vi "Main.vi"(11 "Module Admin":refnum<class "Delacor_lib_QMH_Module Admin.lvclass">) -> ()   [LabVIEW 2024, in "UI.lvlib"]
doc: "This template is based off of the Queued Message Handler design pattern and the Queued Message Handler project template that ships with LabVIEW.\n\nThe main difference is that the queue is private to this module and communication between modules is performed via Broadcast and Request events.\n\nRequest events are wrapped in public API methods and are handled in the Event Handling Loop (EHL) of this VI. Any module can register for Broadcast events sent by this module. The EHL generates messages based on user interface actions.\n\nThe Message Handling Loop (MHL) processes messages generated by the EHL, or by other messages. The messages are string values, so new messages can be added easily to the Message Cases case structure in the MHL. Each message cluster can also provide an optional value for Message Data, which is a variant that can be converted to whatever message-specific data is required.\n_____\nBased on DQMH Project Template 7.0.0.1280."
uses:
  UI.lvlib
  <vilib>/Delacor/Delacor QMH/Libraries/Module Admin_class/Delacor_lib_QMH_Module Admin.lvclass
  Module Data--cluster.ctl
  Ready Drive State Machine.ctl
  Start Ready Drive State Machine (Reply Payload)--cluster.ctl
  <vilib>/Delacor/Delacor QMH/Libraries/Message Queue_class/Delacor_lib_QMH_Message Queue.lvclass/Delacor_lib_QMH_Message Queue.ctl
  Stop Argument--cluster.ctl
  <vilib>/Delacor/Delacor QMH/Libraries/Module Admin_class/Delacor_lib_QMH_Module Admin.lvclass/Delacor_lib_QMH_Module Admin.ctl
  <vilib>/Utility/miscctls.llb/LVPointTypeDef.ctl
  <vilib>/Delacor/Delacor QMH/Libraries/Message Queue_class/Delacor_lib_QMH_Enqueue Message (Single).vi
  <vilib>/Delacor/Delacor QMH/Libraries/Module Admin_class/Delacor_lib_QMH_Get External Launch.vi
  <vilib>/Delacor/Delacor QMH/Libraries/Message Queue_class/Delacor_lib_QMH_Message Queue.lvclass
  Hardware Controller/Hardware Controller.lvlib
  Logger/Logger.lvlib
  Auto Mode/Auto Modo.lvlib
panel:
  in  "Fault Tab Control":enum32{"System Fault"}(tab)
  out "System Fault":bool
  in  "Clear Fault":bool
  in  "Data Tab Control":enum32{"XFL Data"}(tab)
  out "Pump Current RPM":dbl(knob) scale=0.0..1600.0
  out "Turbine Current RPM":dbl(knob) scale=0.0..1600.0 scale format="%#.3g"
  out "Turbine Shaft Torque (Nm)":dbl(knob) scale=0.0..25.0 scale format="%#.3g"
  out "Flow Velocity (m/s)":dbl(knob) scale=0.0..3.0
  out "Temperature (°C)":dbl(knob) scale=10.0..40.0
  out "Pressure Turbine Outlet":dbl(knob) scale=0.0..10.0
  out "Pressure Turbine Inlet":dbl(knob) scale=0.0..10.0
  out "Pressure Pump Outlet":dbl(knob) scale=0.0..10.0
  out "Pressure Pump Inlet":dbl(knob) scale=0.0..10.0
  in  "Logger Tab Control":enum32{"Logger"}(tab)
  in  "Start Logging":bool
  in  "Stop Logging":bool
  in  "Folder Path":path
  out "Logging":bool
  in  "Auto Mode Tab Control":enum32{"Auto Mode"}(tab)
  out "Total Steps":i32
  in  "Start Sequence":bool
  in  "Auto Configuration File":path
  in  "Load Configuration":bool
  out "Pump RPMs":i64[](array[numeric])
  out "Turbine RPMs":i64[](array[numeric])
  out "Duration":i64[](array[numeric])
  out "Current Step":i32
  out "Auto Mode Status":bool
  out "Steps Slide":dbl(slide) scale=0.0..10.0
  out "IOLink System State Out":map{string, dbl}(c390)
  in  "IOLink Connections Tab":enum32{"IOLink Connection"}(tab)
  in  "Close IOLink Connection":bool
  in  "Start IOLink Connection":bool
  out "IOLink Connection Status":bool
  out "error out":errorcluster
  in  "Drive Manual Control":enum32{"Drive Manual Control"}(tab)
  in  "Set Turbine RPM":bool
  out "Pump Ready":bool
  out "Turbine Ready":bool
  out "Pump Actual RPM":dbl
  out "Turbine Actual RPM":dbl
  in  "Pump Target RPM":i16
  in  "Turbine Target RPM":i16
  in  "Set Pump RPM":bool
  in  "Set Both RPM":bool
  in  "Set Ready":bool
  in  "EtherCAT Connections":enum32{"EtherCAT Connections"}(tab)
  out "Attempt EtherCAT Connection":bool
  out "EtherCAT Connection Status":bool
  in  "Start EtherCAT Connection":bool
  in  "Close EtherCAT Connection":bool
  in  "Abort":bool
  out "EtherCAT System State Out":map{string, dbl}(c390)
  out "Status":string
  in  "Simulate MHL Error":bool
  in  "Simulate EHL Error":bool
  # "This template is for the DQMH framework. See the block diagram for more information on how to use this template."
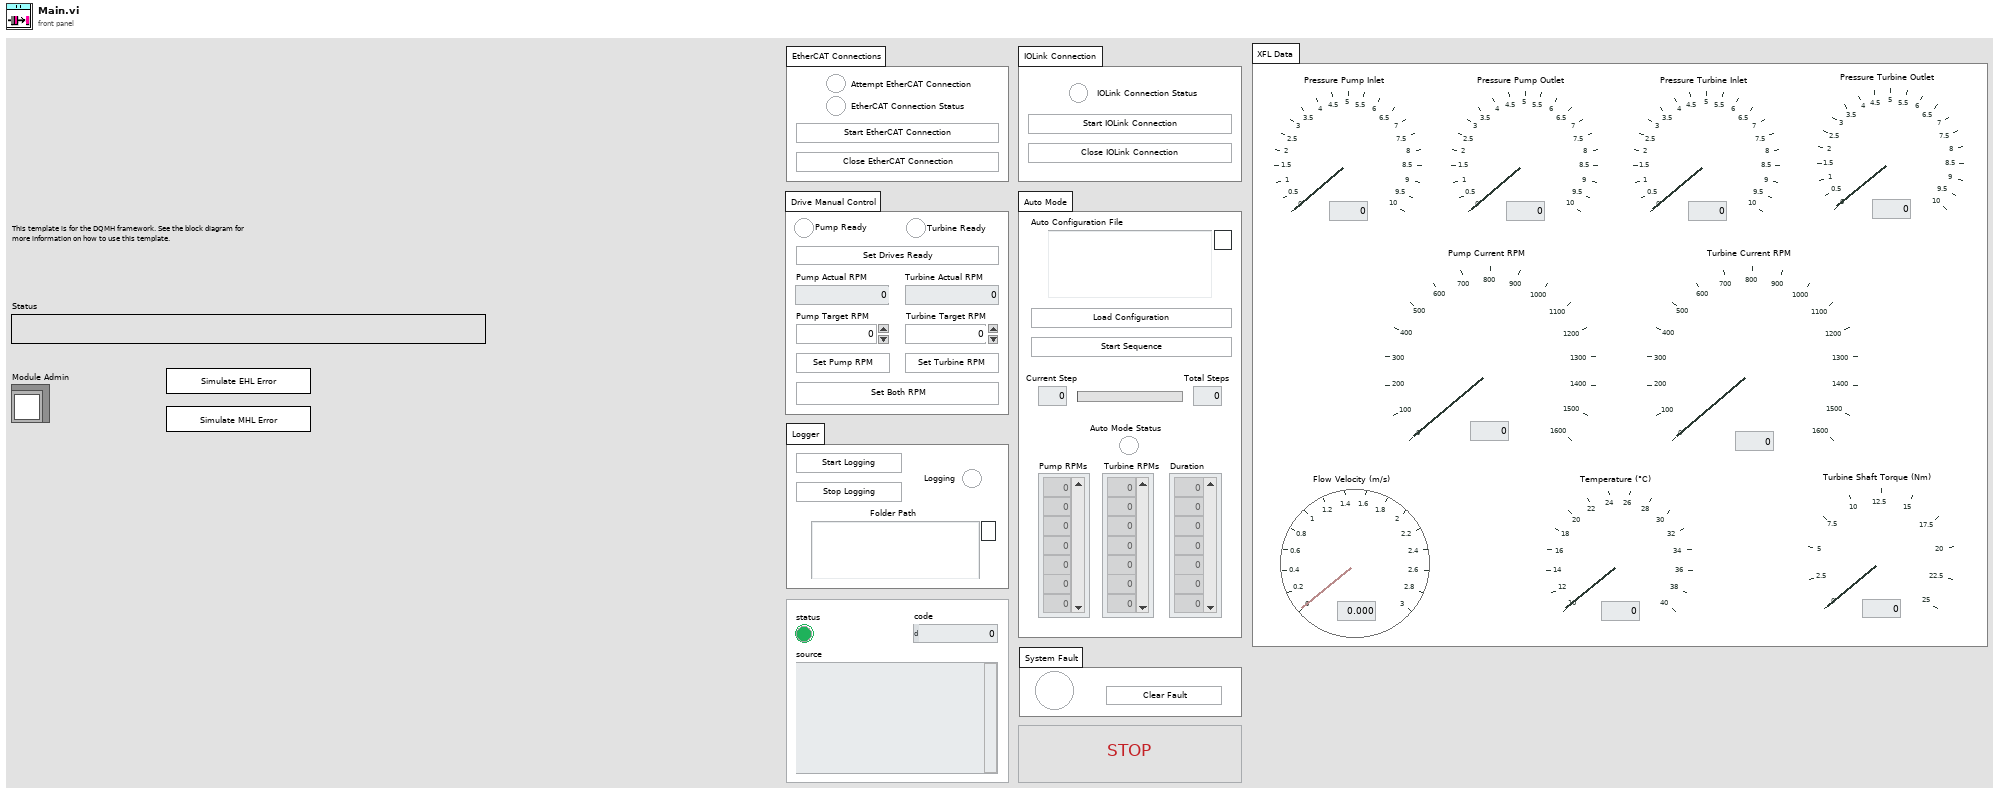
[diagram p1: front panel]
types:
  T1 = typedef "UI.lvlib/Request Events--cluster.ctl" = cluster{"Stop Module":refnum<user-event>, "Show Panel":refnum<user-event>, "Hide Panel":refnum<user-event>, "Get Module Execution Status":refnum<user-event>, "Show Diagram":refnum<user-event>, "Private":cluster{"Launch Hardware Controller":refnum<user-event>, "Register Helper Loop for Hardware Contrller Broadcast":refnum<user-event>, "Start Logger Module":refnum<user-event>, "Start Auto Mode Module":refnum<user-event>}, "Start Ready Drive State Machine":refnum<user-event>}
  T2 = typedef "Logger.lvlib/Broadcast Events--cluster.ctl" = cluster{"Module Did Init":refnum<user-event>, "Status Updated":refnum<user-event>, "Error Reported":refnum<user-event>, "Module Did Stop":refnum<user-event>, "Update Module Execution Status":refnum<user-event>, "Logger Status Updated":refnum<user-event>}
  T3 = typedef "Auto Modo.lvlib/Broadcast Events--cluster.ctl" = cluster{"Module Did Init":refnum<user-event>, "Status Updated":refnum<user-event>, "Error Reported":refnum<user-event>, "Module Did Stop":refnum<user-event>, "Update Module Execution Status":refnum<user-event>, "Current RPM Index":refnum<user-event>, "Auto Mode Status Updated":refnum<user-event>}
  T4 = typedef "Hardware Controller.lvlib/Broadcast Events--cluster.ctl" = cluster{"Module Did Init":refnum<user-event>, "Status Updated":refnum<user-event>, "Error Reported":refnum<user-event>, "Module Did Stop":refnum<user-event>, "Update Module Execution Status":refnum<user-event>, "System State Updated":refnum<user-event>, "EtherCAT Data Updated":refnum<user-event>, "System Fault Updated":refnum<user-event>, "EtherCAT Connection Status Updated":refnum<user-event>, "HardwareController IOLink Data Updated":refnum<user-event>, "IOLink Connection Updated":refnum<user-event>, "HardwareController EtherCAT Data Updated":refnum<user-event>}
  T5 = typedef "UI.lvlib/Ready Drive State Machine.ctl" = cluster{"Wait Notifier":refnum<notifier>, "wait for reply":bool, "Timeout":i32, "State":enum16{"Clear Fault", "Check Fault", "Set Ready to Switch ON", "Check Ready to Switch ON", "Set Switch ON", "Check Switch ON", "Ready Drive Completed"}, "Error":errorcluster}
  T6 = typedef "UI.lvlib/Module Data--cluster.ctl" = cluster{"Status":string, "Pump RPMs":i64[], "Duration":i64[], "Turbine RPMs":i64[]}
  T7 = enum16{"Clear Fault", "Check Fault", "Set Ready to Switch ON", "Check Ready to Switch ON", "Set Switch ON", "Check Switch ON", "Ready Drive Completed"}
  T8 = typedef "UI.lvlib/Start Ready Drive State Machine (Reply Payload)--cluster.ctl" = cluster{"error":errorcluster}
  T9 = enum32{"invalid lock state", "Not Locked", "Locked (No Password)", "Password-protected"}
  T10 = typedef "UI.lvlib/Stop Argument--cluster.ctl" = cluster{"Origin":string, "Exit via Stop Module Req?":bool, "Wait for Module to stop?":bool}
  T11 = typedef "LVPointTypeDef.ctl" = cluster{"Horizontal":i16, "Vertical":i16}
  T12 = enum32{"Invalid", "Standard", "Closed", "Hidden", "Minimized", "Maximized"}
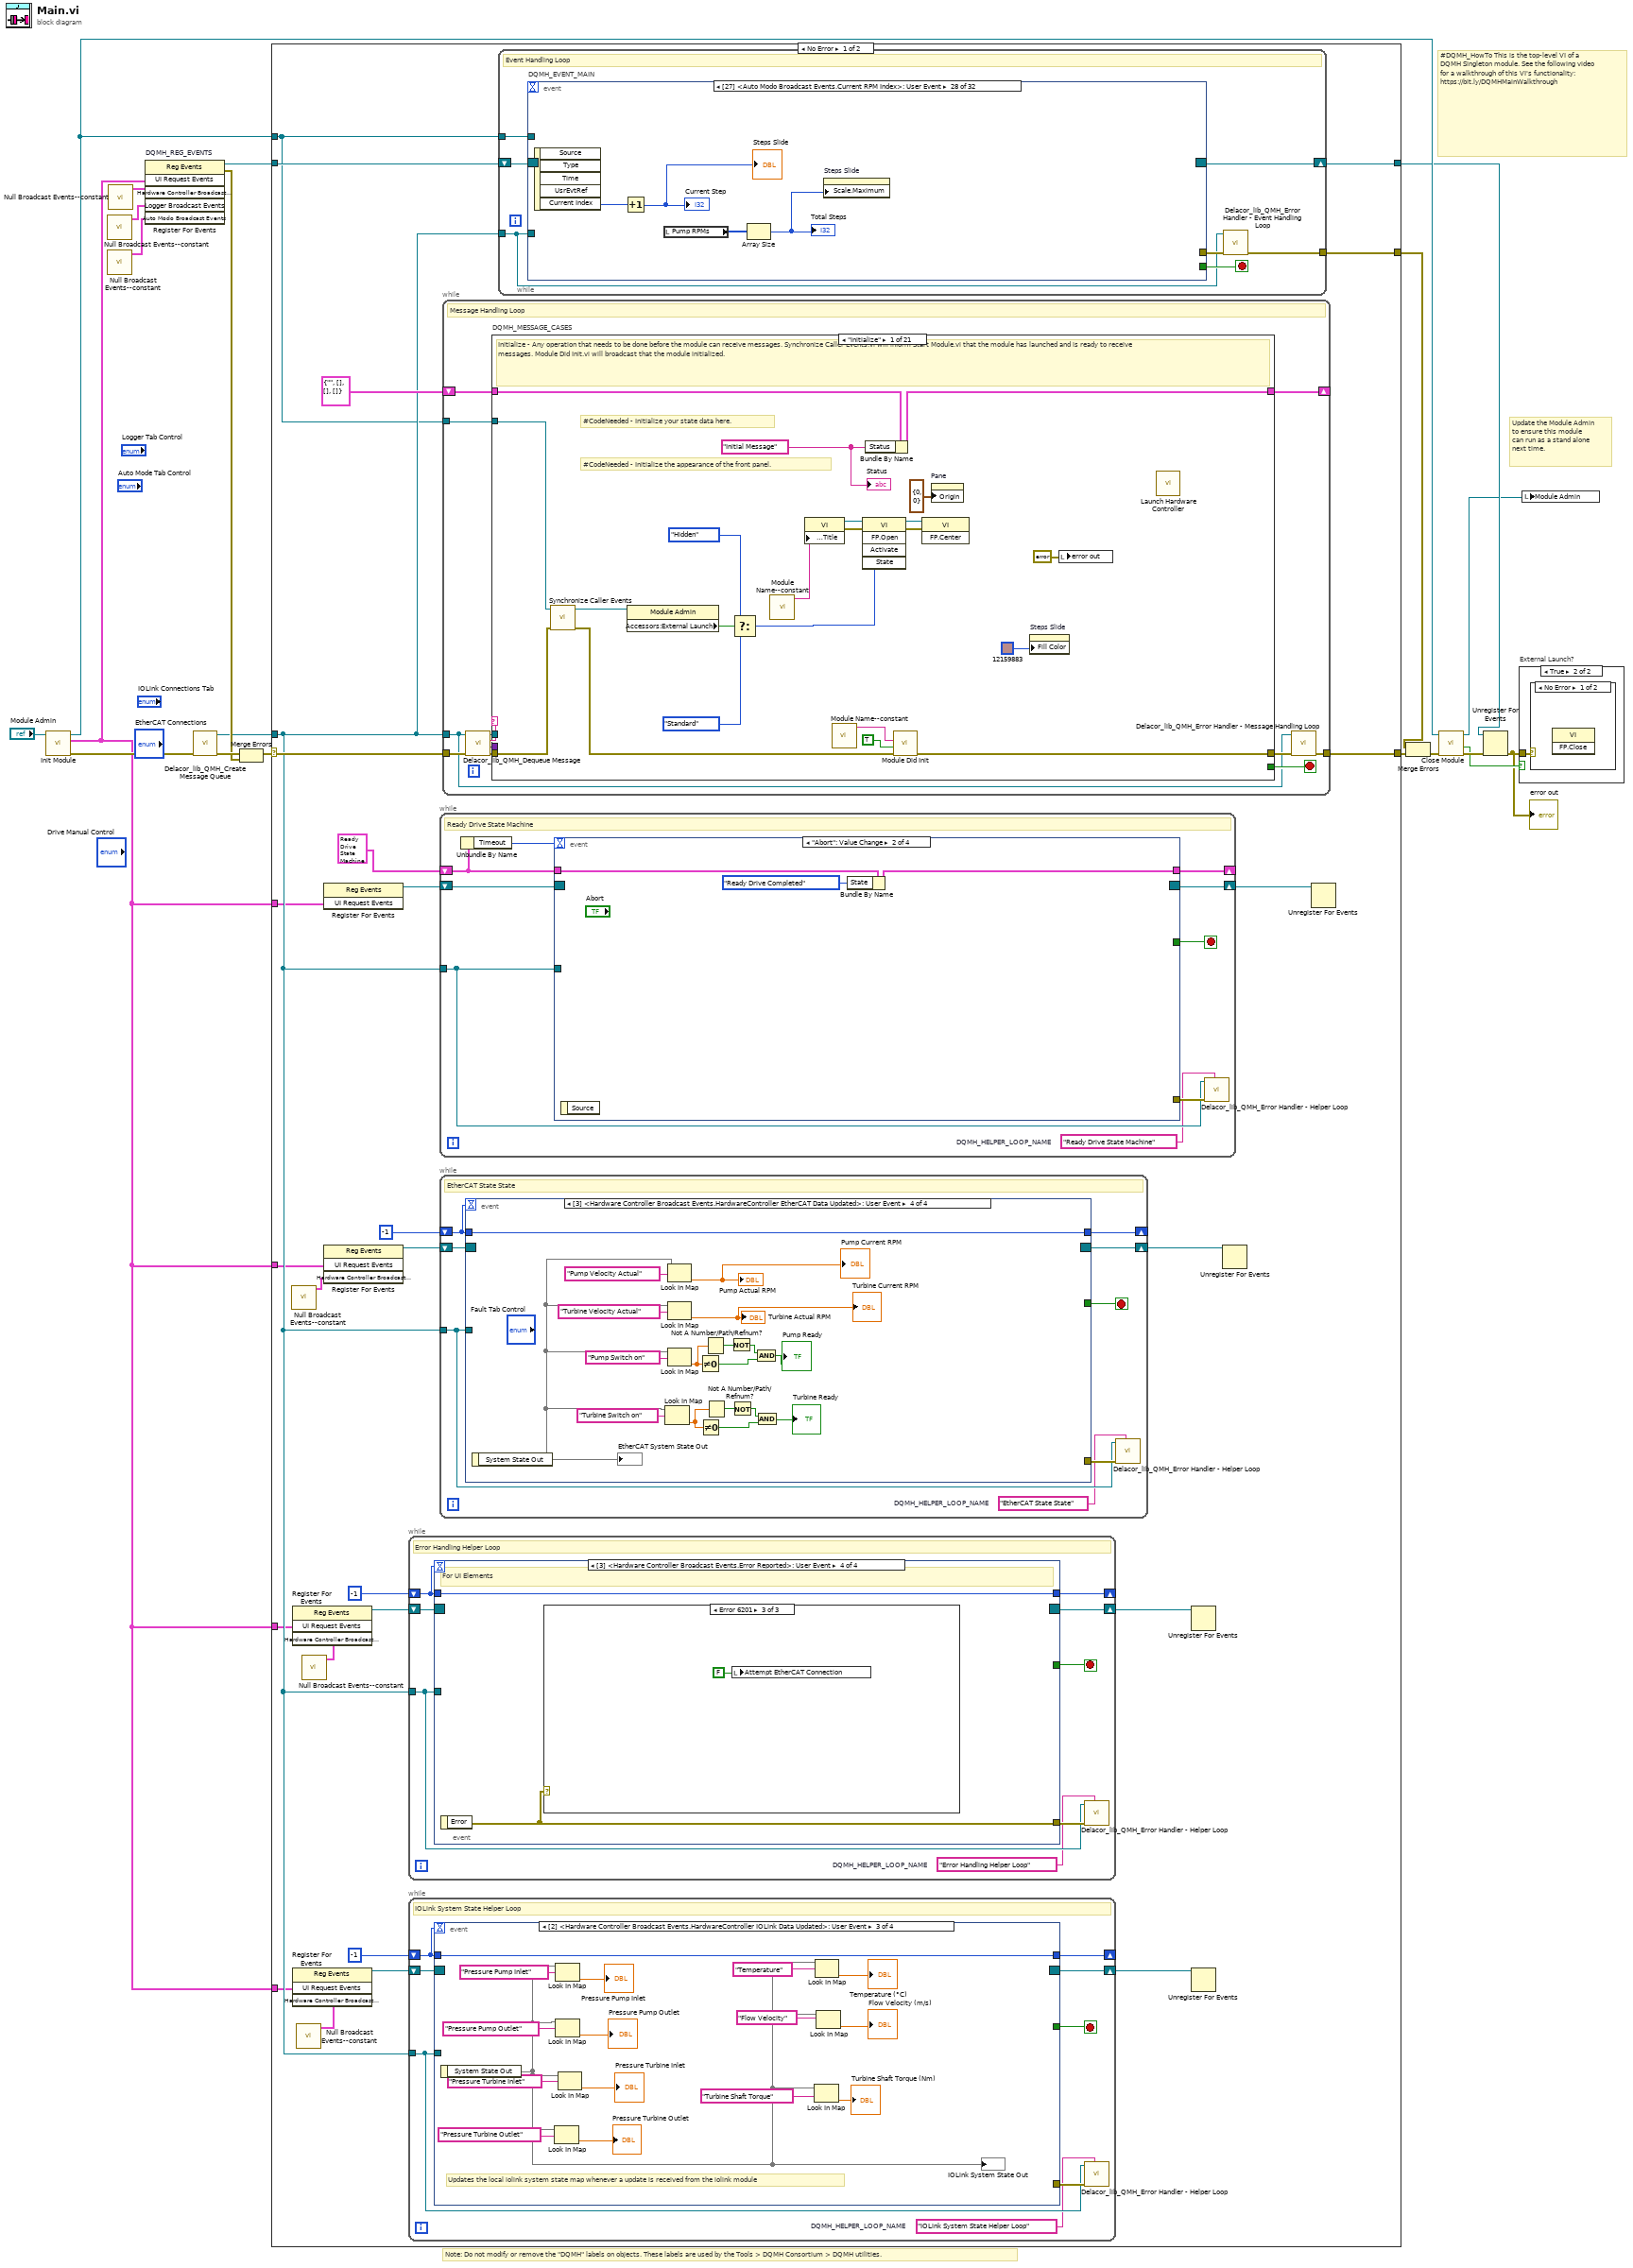
[diagram p0: block diagram]
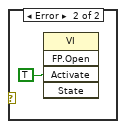
[diagram p3: hidden frame]
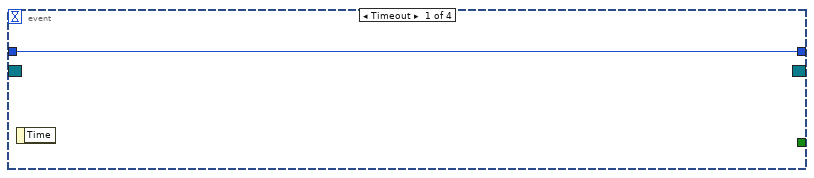
[diagram p4: hidden frame]
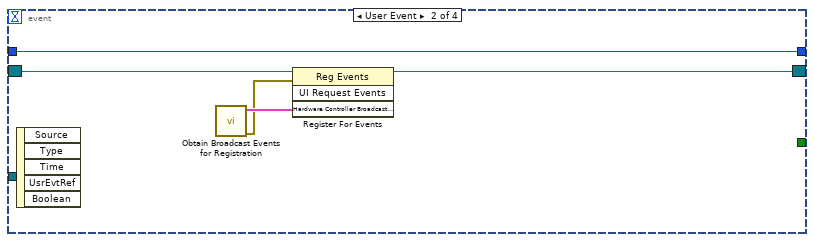
[diagram p5: hidden frame]
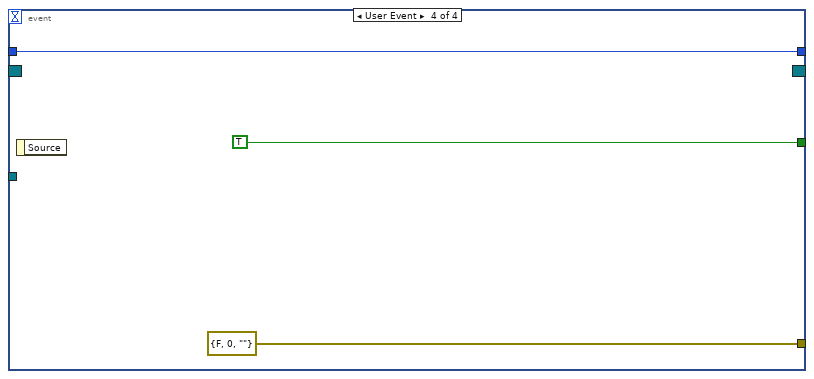
[diagram p6: hidden frame]
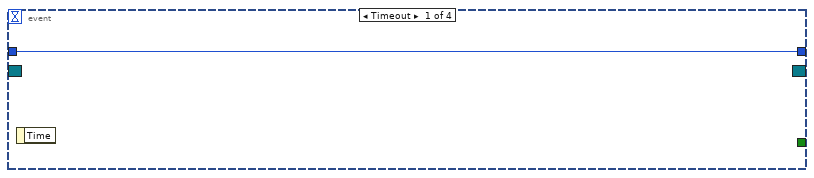
[diagram p7: hidden frame]
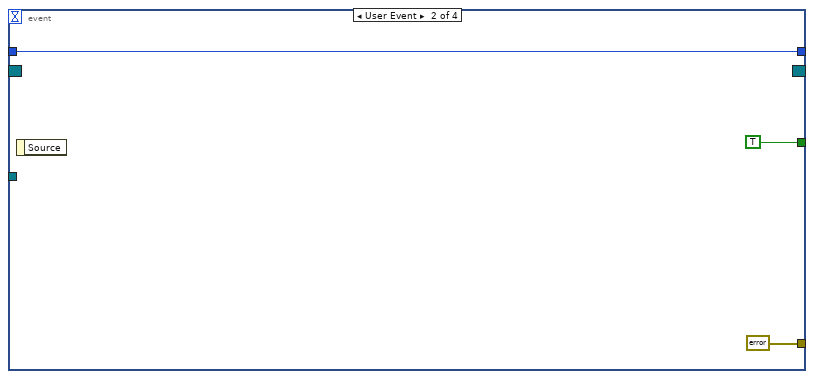
[diagram p8: hidden frame]
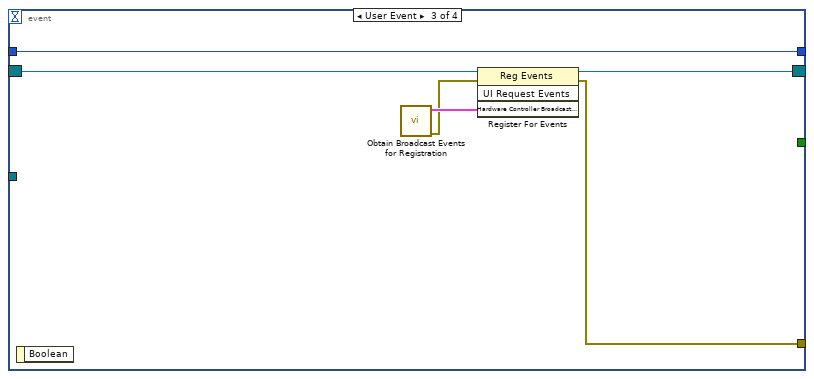
[diagram p9: hidden frame]
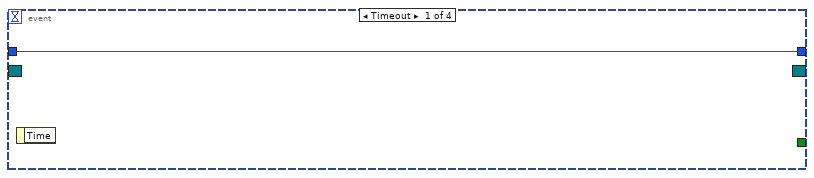
[diagram p12: hidden frame]
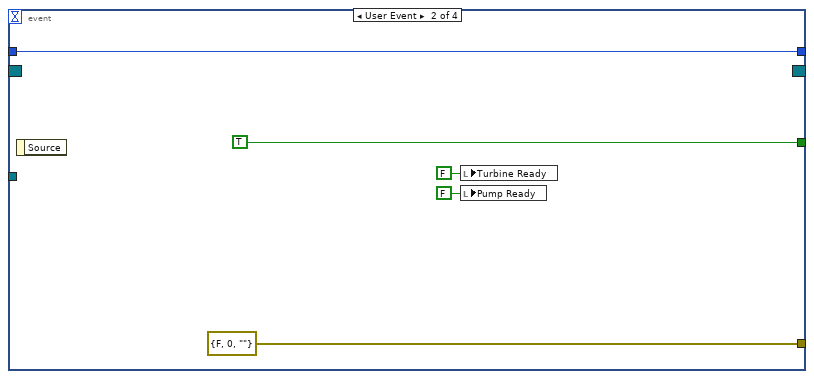
[diagram p13: hidden frame]
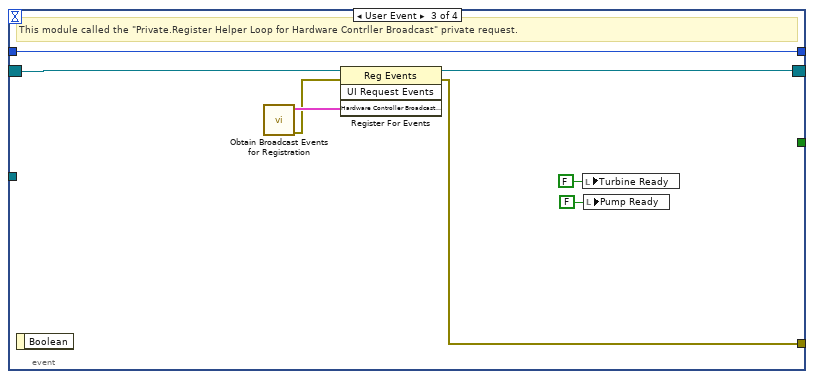
[diagram p14: hidden frame]
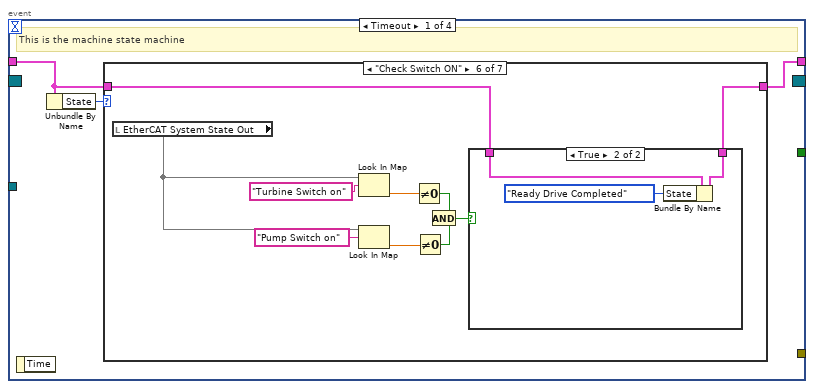
[diagram p15: hidden frame]
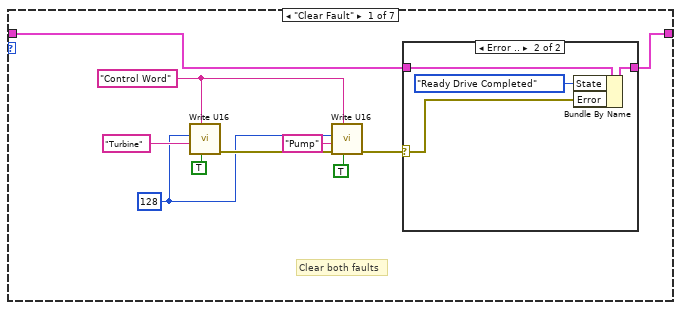
[diagram p16: hidden frame]
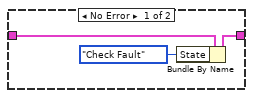
[diagram p17: hidden frame]
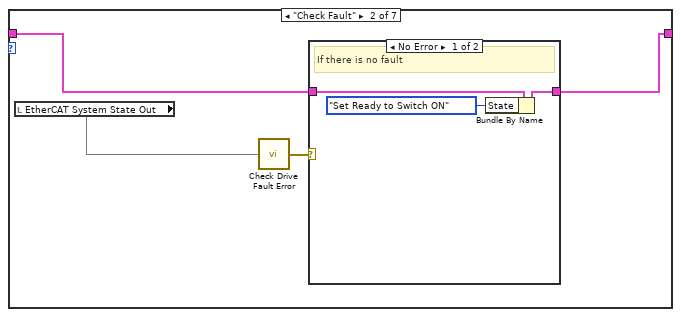
[diagram p18: hidden frame]
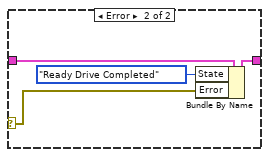
[diagram p19: hidden frame]
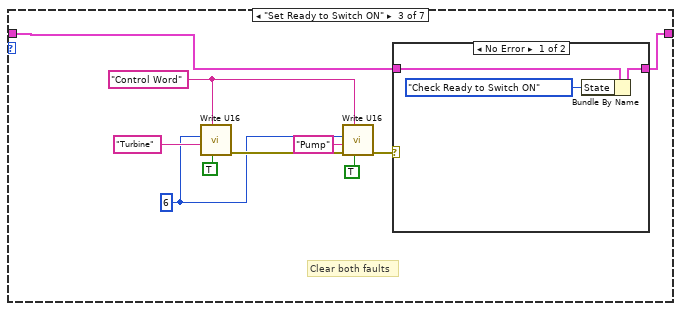
[diagram p20: hidden frame]
diagram:
  # "#DQMH_HowTo This is the top-level VI of a DQMH Singleton module. See the following video for a walkthrough of this VI's functionality: https://bit.ly/DQMHMainWalkthrough"
  # "Note: Do not modify or remove the \"DQMH\" labels on objects. These labels are used by the Tools > DQMH Consortium > DQMH utilities."
  # "Update the Module Admin to ensure this module can run as a stand alone next time."
  n1 = call "Init Module.vi"("Singleton Module Admin in"="Module Admin") -> ("error out"=w19:errorcluster, "UI Request Events"=w3:T1, "Singleton Module Admin out"=w12:refnum<class "Delacor_lib_QMH_Module Admin.lvclass">)  [unwired: 8 in]
  n2 = call "Null Broadcast Events--constant.vi"() -> ("Logger Broadcast Events"=w2:T2)  [unwired: 11 in]
  n3 = call "Null Broadcast Events--constant.vi"() -> ("Auto Modo Broadcast Events"=w1:T3)  [unwired: 11 in]
  n4 = call "Null Broadcast Events--constant.vi"() -> ("Hardware Controller Broadcast Events"=w5:T4)  [unwired: 11 in]
  n5 = register-events "DQMH_REG_EVENTS"(w3, w5, w2, w1) -> (reference out=w10:refnum<event-registration>, error out=w13:errorcluster)  [unwired: 2 in]
  n6 = call <vilib>:"Delacor_lib_QMH_Create Message Queue.vi"("error in"=w19) -> ("error out"=w15:errorcluster, "Message Queue"=w9:refnum<class "Delacor_lib_QMH_Message Queue.lvclass">)  [unwired: 9 in]
  n7 = Merge Errors(w15, w13) -> (w14:errorcluster)
  n8 = case shown="No Error" w14 {
    selector: w14 -> [w45 w626]
    tunnel: [w47 w625] -> w20
    tunnel: [w44 w624] -> w11
    tunnel: w10 -> [w42 w624]
    tunnel: w9 -> [w41 w619]
    tunnel: [w46 _] -> w17
    tunnel: w12 -> [w40 w620]
    tunnel: w3 -> [w39 _]
    tunnel: w3 -> [w35 _]
    tunnel: w3 -> [w30 _]
    tunnel: w3 -> [w25 _]
    frame No Error {
      n9 = call "Null Broadcast Events--constant.vi"() -> ("Hardware Controller Broadcast Events"=w31:T4)  [unwired: 11 in]
      n10 = call "Null Broadcast Events--constant.vi"() -> ("Hardware Controller Broadcast Events"=w21:T4)  [unwired: 11 in]
      n11 = register-events ("DQMH_HELPER_REGFOREVENTS")(w25, w21) -> (reference out=w23:refnum<event-registration>)  [unwired: 2 in, 1 out]
      n12 = call "Null Broadcast Events--constant.vi"() -> ("Hardware Controller Broadcast Events"=w26:T4)  [unwired: 11 in]
      n13 = register-events ("DQMH_HELPER_REGFOREVENTS")(w30, w26) -> (reference out=w28:refnum<event-registration>)  [unwired: 2 in, 1 out]
      n14 = register-events ("DQMH_HELPER_REGFOREVENTS")(w39) -> (reference out=w37:refnum<event-registration>)  [unwired: 2 in, 1 out]
      n15 = register-events ("DQMH_HELPER_REGFOREVENTS")(w35, w31) -> (reference out=w33:refnum<event-registration>)  [unwired: 2 in, 1 out]
      n16 = while "DQMH_HELPER_LOOP" {
        shift-right: [w88] -> _
        shift-left: -1 -> [w87]
        shift-right: [w85] -> w29
        shift-left: w28 -> [w86]
        tunnel: w41 -> [w82]
        stop <- w84 stop-if-true
        w81 = "Error Handling Helper Loop"  # DQMH_HELPER_LOOP_NAME
        # "Error Handling Helper Loop"
        n17 = event "DQMH_HELPER_EVENT_STRUCTURE" shown="[3] <Hardware Controller Broadcast Events.Error Reported>: User Event" {
          selector: w86 -> [_ _ w95 _]
          dyn-events: [_ _ w94 _] -> w85
          timeout: w87 -> [_ _ _ _]
          tunnel: w87 -> [w89 w92 w98 w100]
          tunnel: [w89 w92 w98 w100] -> w88
          tunnel: [_ TRUE _ _] -> w84
          tunnel: [_ errorcluster {"status"=FALSE, "code"=0, "source"=""} ("error constant") w93 w99] -> w83
          tunnel: w82 -> [_ _ _ _]
          event Timeout {
            n18 = event-data() -> ()  [unwired: 1 in, 1 out]
          }
          event User Event {
            n19 = event-data() -> ()  [unwired: 1 in, 1 out]
          }
          event User Event {
            n20 = event-data() -> ()  [unwired: 1 in, 1 out]
            n21 = call "Obtain Broadcast Events for Registration.vi"() -> ("error out"=w96:errorcluster, "Hardware Controller Broadcast Events"=w97:T4)  [unwired: 9 in, 1 out]
            n22 = register-events ("DQMH_HELPER_REGFOREVENTS")(reference=w95, error in=w96, w97) -> (reference out=w94:refnum<event-registration>, error out=w93:errorcluster)  [unwired: 1 in]
          }
          event User Event {
            # "For UI Elements"
            n23 = event-data() -> ("Error"=w99:errorcluster)  [unwired: 1 in]
            n24 = case shown="Error 6201" w99 {
              frame No Error {
              }
              frame Default {
              }
              frame Error {
                n25 = local write "Attempt EtherCAT Connection"(FALSE ("Attempt EtherCAT Connection")) -> ()
              }
            }
          }
        }
        n26 = call-dynamic "Delacor_lib_QMH_Error Handler - Helper Loop.vi"("Error Debug"=w81, "error in"=w83, "Message Queue in"=w82) -> ()  [unwired: 7 in, 2 out]
      }
      n27 = while "DQMH_HELPER_LOOP" {
        shift-right: [w55] -> _
        shift-left: -1 -> [w54]
        shift-right: [w52] -> w24
        shift-left: w23 -> [w53]
        tunnel: w41 -> [w49]
        stop <- w51 stop-if-true
        w48 = "IOLink System State Helper Loop"  # DQMH_HELPER_LOOP_NAME
        # "IOLink System State Helper Loop"
        n28 = event "DQMH_HELPER_EVENT_STRUCTURE" shown="[2] <Hardware Controller Broadcast Events.HardwareController IOLink Data Updated>: User Event" {
          selector: w53 -> [_ w58 _ _]
          dyn-events: [_ w57 _ _] -> w52
          timeout: w54 -> [_ _ _ _]
          tunnel: w54 -> [w56 w61 w77 w80]
          tunnel: [w56 w61 w77 w80] -> w55
          tunnel: [_ _ _ TRUE] -> w51
          tunnel: [_ _ _ errorcluster {"status"=FALSE, "code"=0, "source"=""} ("error constant")] -> w50
          tunnel: w49 -> [_ _ _ _]
          event Timeout {
            n29 = event-data() -> ()  [unwired: 1 in, 1 out]
          }
          event User Event {
            n30 = event-data() -> ()  [unwired: 1 in, 5 out]
            n31 = call "Obtain Broadcast Events for Registration.vi"() -> ("error out"=w59:errorcluster, "Hardware Controller Broadcast Events"=w60:T4)  [unwired: 9 in, 1 out]
            n32 = register-events ("DQMH_HELPER_REGFOREVENTS")(reference=w58, error in=w59, w60) -> (reference out=w57:refnum<event-registration>)  [unwired: 1 in, 1 out]
          }
          event User Event {
            # "Updates the local iolink system state map whenever a update is received from the iolink module"
            n33 = event-data() -> ("System State Out"=w64:map{string, dbl})  [unwired: 1 in]
            "IOLink System State Out" <- w64
            n34 = Look In Map(map=w64, key="Pressure Turbine Outlet") -> (value=→"Pressure Turbine Outlet":dbl)  [unwired: 1 in, 1 out]
            n35 = Look In Map(map=w64, key="Pressure Pump Inlet") -> (value=→"Pressure Pump Inlet":dbl)  [unwired: 1 in, 1 out]
            n36 = Look In Map(map=w64, key="Pressure Pump Outlet") -> (value=→"Pressure Pump Outlet":dbl)  [unwired: 1 in, 1 out]
            n37 = Look In Map(map=w64, key="Pressure Turbine Inlet") -> (value=→"Pressure Turbine Inlet":dbl)  [unwired: 1 in, 1 out]
            n38 = Look In Map(map=w64, key="Turbine Shaft Torque") -> (value=→"Turbine Shaft Torque (Nm)":dbl)  [unwired: 1 in, 1 out]
            n39 = Look In Map(map=w64, key="Temperature") -> (value=→"Temperature (°C)":dbl)  [unwired: 1 in, 1 out]
            n40 = Look In Map(map=w64, key="Flow Velocity") -> (value=→"Flow Velocity (m/s)":dbl)  [unwired: 1 in, 1 out]
          }
          event User Event {
            n41 = event-data() -> ()  [unwired: 1 in, 1 out]
          }
        }
        n42 = call-dynamic "Delacor_lib_QMH_Error Handler - Helper Loop.vi"("Error Debug"=w48, "error in"=w50, "Message Queue in"=w49) -> ()  [unwired: 7 in, 2 out]
      }
      n43 = while "DQMH_HELPER_LOOP" {
        shift-right: [w150] -> _
        shift-left: T5 {"Wait Notifier"=refnum, "wait for reply"=FALSE, "Timeout"=-1, "State"=enum."Clear Fault", "Error"={"status"=FALSE, "code"=0, "source"=""}} ("State Machine States") -> [w143]
        shift-right: [w148] -> w38
        shift-left: w37 -> [w149]
        tunnel: w41 -> [w145]
        stop <- w147 stop-if-true
        w144 = "Ready Drive State Machine"  # DQMH_HELPER_LOOP_NAME
        # "Ready Drive State Machine"
        n44 = Unbundle By Name(w143) -> ("Timeout"=w142:i32)
        n45 = event "DQMH_HELPER_EVENT_STRUCTURE" shown="[1] \"Abort\": Value Change" {
          selector: w149 -> [_ _ _ _]
          dyn-events: [_ _ _ _] -> w148
          timeout: w142 -> [_ _ _ _]
          tunnel: w143 -> [w152 w260 w263 w269]
          tunnel: [w151 w259 w263 w268] -> w150
          tunnel: [_ _ TRUE _] -> w147
          tunnel: [_ _ errorcluster {"status"=FALSE, "code"=0, "source"=""} ("error constant") _] -> w146
          tunnel: w145 -> [_ _ _ _]
          event Timeout {
            # "This is the machine state machine"
            n46 = event-data() -> ()  [unwired: 1 in, 1 out]
            n47 = Unbundle By Name(w152) -> ("State"=w153:T7)
            n48 = case shown="\"Check Switch ON\"" w153 {
              tunnel: w152 -> [w155 w172 w183 w200 w217 w233 w251]
              tunnel: [w154 w171 w182 w199 w216 w232 w249] -> w151
              frame "Clear Fault" {
                w163 = "Control Word" ("Variable")
                w158 = u16 128 ("Data")
                # "Clear both faults"
                n49 = call "Write U16.vi"("wait for reply (T)"=TRUE, "Variable"=w163, "Drive"="Turbine", "Data"=w158) -> ("error out"=w161:errorcluster)  [unwired: 6 in, 1 out]
                n50 = call "Write U16.vi"("wait for reply (T)"=TRUE, "Variable"=w163, "error in"=w161, "Drive"="Pump", "Data"=w158) -> ("error out"=w156:errorcluster)  [unwired: 5 in, 1 out]
                n51 = case shown="Error .." w156 {
                  selector: w156 -> [_ w167]
                  tunnel: w155 -> [w166 w170]
                  tunnel: [w165 w169] -> w154
                  frame No Error {
                    n52 = Bundle By Name(cluster=w166, "State"=T7."Check Fault") -> (w165:T5)
                  }
                  frame Error {
                    n53 = Bundle By Name(cluster=w170, "State"=T7."Ready Drive Completed", "Error"=w167) -> (w169:T5)
                  }
                }
              }
              frame "Check Fault" {
                n54 = local read "EtherCAT System State Out"() -> (w174:map{string, dbl})
                n55 = call "Check Drive Fault Error.vi"("Map"=w174) -> ("error out"=w173:errorcluster)
                n56 = case shown="No Error" w173 {
                  selector: w173 -> [_ w178]
                  tunnel: w172 -> [w177 w180]
                  tunnel: [w176 w179] -> w171
                  frame No Error {
                    # "If there is no fault"
                    n57 = Bundle By Name(cluster=w177, "State"=T7."Set Ready to Switch ON") -> (w176:T5)
                  }
                  frame Error {
                    n58 = Bundle By Name(cluster=w180, "State"=T7."Ready Drive Completed", "Error"=w178) -> (w179:T5)
                  }
                }
              }
              frame "Set Ready to Switch ON" {
                w191 = "Control Word" ("Variable")
                w186 = u16 6 ("Data")
                # "Clear both faults"
                n59 = call "Write U16.vi"("wait for reply (T)"=TRUE, "Variable"=w191, "Drive"="Turbine", "Data"=w186) -> ("error out"=w189:errorcluster)  [unwired: 6 in, 1 out]
                n60 = call "Write U16.vi"("wait for reply (T)"=TRUE, "Variable"=w191, "error in"=w189, "Drive"="Pump", "Data"=w186) -> ("error out"=w184:errorcluster)  [unwired: 5 in, 1 out]
                n61 = case shown="No Error" w184 {
                  selector: w184 -> [_ w195]
                  tunnel: w183 -> [w194 w198]
                  tunnel: [w193 w197] -> w182
                  frame No Error {
                    n62 = Bundle By Name(cluster=w194, "State"=T7."Check Ready to Switch ON") -> (w193:T5)
                  }
                  frame Error {
                    n63 = Bundle By Name(cluster=w198, "State"=T7."Ready Drive Completed", "Error"=w195) -> (w197:T5)
                  }
                }
              }
              frame "Check Ready to Switch ON" {
                n64 = local read "EtherCAT System State Out"() -> (w202:map{string, dbl})
                n65 = Look In Map(map=w202, key="Turbine Ready to switch on") -> (value=w206:dbl)  [unwired: 1 in, 1 out]
                n66 = Look In Map(map=w202, key="Pump Ready to switch on") -> (value=w205:dbl)  [unwired: 1 in, 1 out]
                n67 = Not Equal To 0?(x=w206) -> (x != 0?=w204:bool)
                n68 = Not Equal To 0?(x=w205) -> (x != 0?=w203:bool)
                n69 = And(x=w204, y=w203) -> (x .and. y?=w201:bool)
                n70 = case shown="True" w201 {
                  tunnel: w200 -> [w210 w214]
                  tunnel: [w209 w213] -> w199
                  frame False {
                    n71 = Bundle By Name(cluster=w210, "State"=T7."Check Ready to Switch ON") -> (w209:T5)
                  }
                  frame True {
                    n72 = Bundle By Name(cluster=w214, "State"=T7."Set Switch ON") -> (w213:T5)
                  }
                }
              }
              frame "Set Switch ON" {
                w224 = "Control Word" ("Variable")
                w219 = u16 7 ("Data")
                n73 = call "Write U16.vi"("wait for reply (T)"=TRUE, "Variable"=w224, "Drive"="Turbine", "Data"=w219) -> ("error out"=w222:errorcluster)  [unwired: 6 in, 1 out]
                n74 = call "Write U16.vi"("wait for reply (T)"=TRUE, "Variable"=w224, "error in"=w222, "Drive"="Pump", "Data"=w219) -> ("error out"=w215:errorcluster)  [unwired: 5 in, 1 out]
                n75 = case shown="No Error" w215 {
                  selector: w215 -> [_ w228]
                  tunnel: w217 -> [w227 w231]
                  tunnel: [w226 w230] -> w216
                  frame No Error {
                    n76 = Bundle By Name(cluster=w227, "State"=T7."Check Switch ON") -> (w226:T5)
                  }
                  frame Error {
                    n77 = Bundle By Name(cluster=w231, "State"=T7."Ready Drive Completed", "Error"=w228) -> (w230:T5)
                  }
                }
              }
              frame "Check Switch ON" {
                n78 = local read "EtherCAT System State Out"() -> (w237:map{string, dbl})
                n79 = Look In Map(map=w237, key="Turbine Switch on") -> (value=w241:dbl)  [unwired: 1 in, 1 out]
                n80 = Look In Map(map=w237, key="Pump Switch on") -> (value=w240:dbl)  [unwired: 1 in, 1 out]
                n81 = Not Equal To 0?(x=w241) -> (x != 0?=w239:bool)
                n82 = Not Equal To 0?(x=w240) -> (x != 0?=w238:bool)
                n83 = And(x=w239, y=w238) -> (x .and. y?=w236:bool)
                n84 = case shown="True" w236 {
                  tunnel: w233 -> [w243 w247]
                  tunnel: [w242 w246] -> w232
                  frame False {
                    n85 = Bundle By Name(cluster=w243, "State"=T7."Check Switch ON") -> (w242:T5)
                  }
                  frame True {
                    n86 = Bundle By Name(cluster=w247, "State"=T7."Ready Drive Completed") -> (w246:T5)
                  }
                }
              }
              frame "Ready Drive Completed", Default {
                n87 = Unbundle By Name(w251) -> ("Error"=w250:errorcluster, "Wait Notifier"=w253:refnum<notifier>, "wait for reply"=w252:bool)
                n88 = Bundle By Name(cluster=w251, "Timeout"=-1) -> (w249:T5)
                n89 = Bundle By Name(cluster=T8 {"error"={"status"=FALSE, "code"=0, "source"=""}} ("Start Ready Drive State Machine (Reply Payload)"), "error"=w250) -> (w255:T8)
                n90 = case "DQMH_FIRE_NOTIFIER" shown="True" w252 {
                  tunnel: w253 -> [_ w257]
                  tunnel: w255 -> [_ w256]
                  frame False {
                  }
                  frame True {
                    n91 = Send Notification(notification=w256, notifier=w257) -> ()  [unwired: 1 in, 2 out]
                  }
                }
              }
            }
          }
          event "Abort": Value Change {
            n92 = event-data() -> ()  [unwired: 1 in, 1 out]
            n93 = Bundle By Name(cluster=w260, "State"=T7."Ready Drive Completed") -> (w259:T5)
          }
          event User Event {
            n94 = event-data() -> ()  [unwired: 1 in, 1 out]
          }
          event User Event {
            # "This start the state machine by going to clear fault state"
            # "Another Module called the \"Start Ready Drive State Machine\" API Method."
            n95 = event-data() -> ("Wait Notifier"=w267:refnum<notifier>, "wait for reply"=w266:bool)  [unwired: 1 in]
            n96 = Bundle By Name(cluster=w269, "Wait Notifier"=w267, "wait for reply"=w266, "Timeout"=10, "State"=T7."Clear Fault") -> (w268:T5)
          }
        }
        n97 = call-dynamic "Delacor_lib_QMH_Error Handler - Helper Loop.vi"("Error Debug"=w144, "error in"=w146, "Message Queue in"=w145) -> ()  [unwired: 7 in, 2 out]
      }
      n98 = while "DQMH_HELPER_LOOP" {
        shift-right: [w109] -> _
        shift-left: -1 -> [w108]
        shift-right: [w106] -> w34
        shift-left: w33 -> [w107]
        tunnel: w41 -> [w103]
        stop <- w105 stop-if-true
        w102 = "EtherCAT State State"  # DQMH_HELPER_LOOP_NAME
        # "EtherCAT State State"
        n99 = event "DQMH_HELPER_EVENT_STRUCTURE" shown="[3] <Hardware Controller Broadcast Events.HardwareController EtherCAT Data Updated>: User Event" {
          selector: w107 -> [_ _ w122 _]
          dyn-events: [_ _ w121 _] -> w106
          timeout: w108 -> [_ _ _ _]
          tunnel: w108 -> [w110 w115 w123 w141]
          tunnel: [w110 w115 w123 w141] -> w109
          tunnel: [_ TRUE _ _] -> w105
          tunnel: [_ errorcluster {"status"=FALSE, "code"=0, "source"=""} ("error constant") w118 _] -> w104
          tunnel: w103 -> [_ _ _ _]
          event Timeout {
            n100 = event-data() -> ()  [unwired: 1 in, 1 out]
          }
          event User Event {
            n101 = event-data() -> ()  [unwired: 1 in, 1 out]
            n102 = local write "Turbine Ready"(FALSE ("Turbine Ready")) -> ()
            n103 = local write "Pump Ready"(FALSE ("Pump Ready")) -> ()
          }
          event User Event {
            # "This module called the \"Private.Register Helper Loop for Hardware Contrller Broadcast\" private request."
            n104 = event-data() -> ()  [unwired: 1 in, 1 out]
            n105 = call "Obtain Broadcast Events for Registration.vi"() -> ("error out"=w119:errorcluster, "Hardware Controller Broadcast Events"=w120:T4)  [unwired: 9 in, 1 out]
            n106 = register-events ("DQMH_HELPER_REGFOREVENTS")(reference=w122, error in=w119, w120) -> (reference out=w121:refnum<event-registration>, error out=w118:errorcluster)  [unwired: 1 in]
            n107 = local write "Turbine Ready"(FALSE ("Turbine Ready")) -> ()
            n108 = local write "Pump Ready"(FALSE ("Pump Ready")) -> ()
          }
          event User Event {
            n109 = event-data() -> ("System State Out"=w136:map{string, dbl})  [unwired: 1 in]
            "EtherCAT System State Out" <- w136
            n110 = Look In Map(map=w136, key="Turbine Switch on") -> (value=w127:dbl)  [unwired: 1 in, 1 out]
            n111 = Look In Map(map=w136, key="Pump Velocity Actual") -> (value=→"Pump Actual RPM" →"Pump Current RPM":dbl)  [unwired: 1 in, 1 out]
            n112 = Look In Map(map=w136, key="Turbine Velocity Actual") -> (value=→"Turbine Actual RPM" →"Turbine Current RPM":dbl)  [unwired: 1 in, 1 out]
            n113 = Look In Map(map=w136, key="Pump Switch on") -> (value=w135:dbl)  [unwired: 1 in, 1 out]
            n114 = Not Equal To 0?(x=w135) -> (x != 0?=w132:bool)
            n115 = Not Equal To 0?(x=w127) -> (x != 0?=w128:bool)
            n116 = Not A Number/Path/Refnum?(number/path/refnum=w135) -> (NaN/Path/Refnum?=w134:bool)
            n117 = Not A Number/Path/Refnum?(number/path/refnum=w127) -> (NaN/Path/Refnum?=w130:bool)
            n118 = Not(x=w134) -> (.not. x?=w133:bool)
            n119 = Not(x=w130) -> (.not. x?=w129:bool)
            n120 = And(x=w133, y=w132) -> (x .and. y?=→"Pump Ready":bool)
            n121 = And(x=w129, y=w128) -> (x .and. y?=→"Turbine Ready":bool)
          }
        }
        n122 = call-dynamic "Delacor_lib_QMH_Error Handler - Helper Loop.vi"("Error Debug"=w102, "error in"=w104, "Message Queue in"=w103) -> ()  [unwired: 7 in, 2 out]
      }
      n123 = while {
        tunnel: w41 -> [w401]
        shift-right: [w407] -> _
        shift-left: T6 {"Status"="", "Pump RPMs"=[], "Duration"=[], "Turbine RPMs"=[]} ("Data Cluster") -> [w408]
        tunnel: w45 -> [w411]
        tunnel: [w409] -> w47
        tunnel: w40 -> [w402]
        stop <- w406 stop-if-true
        # "Message Handling Loop"
        n124 = call-dynamic "Delacor_lib_QMH_Dequeue Message.vi"("error in"=w411, "Message Queue in"=w401) -> ("error out"=w410:errorcluster, "Message Data"=w404:variant, "Message"=w405:string, "Message Queue out"=w403:refnum<class "Delacor_lib_QMH_Message Queue.lvclass">)  [unwired: 6 in]
        n125 = case "DQMH_MESSAGE_CASES" shown="\"Initialize\"" w405 {
          selector: w405 -> [_ _ _ _ _ _ _ _ _ _ _ _ _ _ _ _ _ _ _ _ w614]
          tunnel: w403 -> [_ _ _ _ _ _ _ _ _ _ _ _ w506 _ _ _ _ w592 _ _ _]
          tunnel: w410 -> [w432 _ w444 w461 w464 w469 w476 w480 w483 w490 w494 w503 w513 w527 w540 w556 w573 w598 w601 w608 w617]
          tunnel: [w430 w435 w445 w461 w463 w468 w475 w480 w483 w491 w494 w502 w509 w527 w540 w556 w573 w593 w600 w608 w618] -> w412
          tunnel: w408 -> [w421 w440 w442 w460 w462 w467 w474 w479 w482 w492 w493 w500 w508 w526 w539 w555 w572 w591 w603 w607 w615]
          tunnel: [w420 w440 w442 w460 w462 w467 w474 w479 w482 w487 w493 w500 w508 w526 w539 w555 w572 w591 w603 w607 w615] -> w407
          tunnel: [_ _ _ _ _ _ _ _ _ _ _ _ _ _ _ _ _ w590 _ _ _] -> w406
          tunnel: w404 -> [_ _ _ _ _ _ _ _ _ _ _ _ w507 _ _ _ _ w589 _ _ _]
          tunnel: w402 -> [w422 _ _ _ _ _ _ _ _ _ _ _ _ _ _ _ _ w584 _ _ _]
          frame "Initialize" {
            w416 = "Initial Message" ("Initial Message")
            # "#CodeNeeded - Initialize the appearance of the front panel."
            # "#CodeNeeded - Initialize your state data here."
            # "Initialize - Any operation that needs to be done before the module can receive messages. Synchronize Caller Events.vi will inform Start Module.vi that the module has launched and is ready to receive messages. Module Did Init.vi will broadcast that the module initialized."
            n126 = call "Synchronize Caller Events.vi"("error in"=w432, "Singleton Module Admin in"=w422) -> ("error out"=w431:errorcluster, "Singleton Module Admin out"=w417:refnum<class "Delacor_lib_QMH_Module Admin.lvclass">)  [unwired: 8 in]
            n127 = property class="Module Admin"(reference=w417) -> ("Accessors:External Launch"=w426:bool)  [unwired: 1 in, 2 out]
            n128 = Select(t=T12."Hidden" ("State"), s=w426, f=T12."Standard" ("State")) -> (s? t:f=w423:T12)
            n129 = call "Module Name--constant.vi"() -> ("Module Name"=w429:string)  [unwired: 11 in]
            n130 = property class="VI"("Front Panel.Title"=w429) -> (reference out=w428:refnum<vi>, error out=w434:errorcluster)  [unwired: 2 in]
            n131 = call "Module Name--constant.vi"() -> ("Module Name"=w418:string)  [unwired: 11 in]
            n132 = invoke class="VI" method="FP.Open"(reference=w428, error in=w434, "State"=w423) -> (reference out=w427:refnum<vi>, error out=w433:errorcluster)  [unwired: 2 in, 3 out]
            n133 = Bundle By Name(cluster=w421, "Status"=w416) -> (w420:T6)
            n134 = call "Module Did Init.vi"("error in"=w431, "Initialized?"=TRUE, "Origin"=w418) -> ("error out"=w430:errorcluster)  [unwired: 8 in]
            n135 = invoke class="VI" method="FP.Center"(reference=w427, error in=w433) -> ()  [unwired: 1 in, 3 out]
            n136 = property on="Pane" class="Pane"("Origin"=T11 {"Horizontal"=0, "Vertical"=0}) -> ()  [unwired: 2 in, 2 out]
            n137 = property on="Steps Slide" class="Slide (strict)"("Fill Color"=u32 12159883) -> ()  [unwired: 2 in, 2 out]
            n138 = local write "error out"(errorcluster {"status"=FALSE, "code"=0, "source"=""} ("error out")) -> ()
            n139 = call "Launch Hardware Controller.vi"() -> ()  [unwired: 11 in, 1 out]
            "Status" <- w416
          }
          frame "Setup Hardware Controller" {
            n140 = call "Register Helper Loop for Hardware Contrller Broadcast.vi"() -> ("error out"=w439:errorcluster)  [unwired: 11 in]
            n141 = call "Launch all Hardware.vi"("error in"=w439) -> ("error out"=w437:errorcluster)  [unwired: 9 in, 1 out]
            n142 = call "Start Logger Module.vi"("error in"=w437) -> ("error out"=w436:errorcluster)  [unwired: 10 in]
            n143 = call "Start Auto Mode Module.vi"("error in"=w436) -> ("error out"=w435:errorcluster)  [unwired: 10 in]
            "Attempt EtherCAT Connection" <- TRUE ("Attempt EtherCAT Connection")
          }
          frame "Start Auto Mode Sequence" {
            n144 = local read "System Fault"() -> (w441:bool)
            n145 = case shown="False" w441 {
              tunnel: [w451 w459] -> w443
              frame False {
                n146 = local read "Auto Configuration File"() -> (w446:path)
                n147 = local read "Folder Path"() -> (w450:path)
                n148 = call <vilib>:"Is Path and Not Empty.vi"("path"=w446) -> ("Is Path and Not Empty?"=w447:bool)  [unwired: 4 in]
                n149 = call <vilib>:"Is Path and Not Empty.vi"("path"=w450) -> ("Is Path and Not Empty?"=w449:bool)  [unwired: 4 in]
                n150 = And(x=w447, y=w449) -> (x .and. y?=w448:bool)
                n151 = case shown="True" w448 {
                  tunnel: [w452 w457] -> w451
                  tunnel: w446 -> [_ w456]
                  frame False {
                    n152 = call "Necessary Files Not Given 7103--error.vi"() -> ("error out"=w452:errorcluster)  [unwired: 11 in]
                  }
                  frame True {
                    n153 = call "LoadAutoConfig.vi"("file path (dialog if empty)"=w456) -> ("Times"=w454:i64[], "Turbine RPMs"=w453:i64[], "Pump RPMs"=w455:i64[])  [unwired: 7 in, 1 out]
                    n154 = local write "Pump RPMs"(w455) -> ()
                    n155 = local write "Turbine RPMs"(w453) -> ()
                    n156 = local write "Duration"(w454) -> ()
                    n157 = local read "Folder Path"() -> (w458:path)
                    n158 = call "Start Sequence.vi"("Folder Path"=w458, "Turbine RPM Array"=w453, "Pump RPM Array"=w455, "Duration (Seconds)"=w454) -> ("error out"=w457:errorcluster)  [unwired: 6 in, 1 out]
                  }
                }
              }
              frame True {
                n159 = call "Fault Exists Cannot start Auto 7102--error.vi"() -> ("error out"=w459:errorcluster)  [unwired: 11 in]
              }
            }
            n160 = Merge Errors(w443, w444) -> (w445:errorcluster)
          }
          frame "---Module Specific---" {
            # "Separator -- The following cases handle messages specific to this Module."
          }
          frame "---Copy This Frame---" {
            # "Duplicate this frame when creating new messages.  Change this comment in the duplicated frame to describe this message."
            n161 = Merge Errors(w464) -> (w463:errorcluster)
          }
          frame "Get Drive Ready" {
            # "Check auto is not \nrunning"
            # "Duplicate this frame when creating new messages.  Change this comment in the duplicated frame to describe this message."
            n162 = call "Check Idle State.vi"() -> ("Idle"=w465:bool)  [unwired: 9 in, 2 out]
            n163 = case shown="True" w465 {
              tunnel: [_ w470] -> w466
              frame False {
              }
              frame True {
                n164 = call "Start Ready Drive State Machine.vi"("wait for reply (T)"=FALSE) -> ("error out"=w470:errorcluster)  [unwired: 9 in, 1 out]
              }
            }
            n165 = Merge Errors(w466, w469) -> (w468:errorcluster)
          }
          frame "Start EtherCAT Connection" {
            # "Call Start EtherCAT connection request and indicates trying connection."
            n166 = local read "EtherCAT Connection Status"() -> (w472:bool)
            n167 = call "Start EtherCAT Conection.vi"("wait for reply (T)"=FALSE) -> ()  [unwired: 9 in, 2 out]
            n168 = case shown="False" w472 {
              frame False {
                n169 = local write "Attempt EtherCAT Connection"(TRUE ("Attempt EtherCAT Connection")) -> ()
              }
              frame True {
              }
            }
            n170 = Merge Errors(w476) -> (w475:errorcluster)
          }
          frame "Start IOLink Connection" {
            # "Call Start EtherCAT connection request and indicates trying connection."
            n171 = call "Start IOLink Connection.vi"("wait for reply (T)"=FALSE) -> ()  [unwired: 9 in, 2 out]
          }
          frame "Close IOLink Connection" {
            n172 = call "Close IOLink Connection.vi"("wait for reply (T)"=FALSE) -> ()  [unwired: 9 in, 2 out]
          }
          frame "Load Auto Configuration" {
            # "Loads the rpms and times for the auto sequence"
            n173 = call "LoadAutoConfig.vi"("file path (dialog if empty)"="Auto Configuration File") -> ("error out"=w489:errorcluster, "Times"=w484:i64[], "Turbine RPMs"=w485:i64[], "Pump RPMs"=w486:i64[])  [unwired: 7 in]
            "Pump RPMs" <- w486
            "Turbine RPMs" <- w485
            "Duration" <- w484
            n174 = Merge Errors(w489, w490) -> (w491:errorcluster)
            n175 = Bundle By Name(cluster=w492, "Pump RPMs"=w486, "Turbine RPMs"=w485, "Duration"=w484) -> (w487:T6)
          }
          frame "---Exit and Error Handling---" {
            # "Separator - The following cases handle errors and exit messages."
          }
          frame "Simulate MHL Error" {
            # "#DQMH_HowTo The 'Simulate MHL Error' button  illustrates how the MHL handles errors. This event is instructional in nature and can be removed."
            # "Simulate an error occurring at the MHL"
            n176 = call "Module Name--constant.vi"() -> ("Module Name"=w496:string)  [unwired: 11 in]
            n177 = Format Into String(format string="Simulated error originating at Message Handling Loop in %s", w496) -> (resulting string=w497:string)  [unwired: 2 in, 1 out]
            n178 = call <vilib>:"Error Cluster From Error Code.vi"("show call chain? (False)"=TRUE, "error message (\"\")"=w497, "error code (0)"=5001) -> ("error out"=w501:errorcluster)  [unwired: 6 in]
            n179 = Merge Errors(w503, w501) -> (w502:errorcluster)
          }
          frame "Error" {
            # "Error - Check the error message data and respond accordingly. This message is sent by the \"Error Handler\" VIs at the end of each loop in this application."
            n180 = Variant To Data(error in=w513, type=errorcluster {"status"=FALSE, "code"=0, "source"=""} ("error constant"), Variant=w507) -> (data=w504:errorcluster, error out=w511:errorcluster)
            n181 = local write "error out"(w504) -> ()
            n182 = call "Error Reported.vi"("Error"=w504) -> ()  [unwired: 10 in, 1 out]
            n183 = case shown="True" TRUE {
              tunnel: [w518 _] -> w510
              tunnel: w506 -> [w516 _]
              tunnel: w504 -> [w517 _]
              frame False {
                n184 = disable-structure shown="Default" {
                  disable-tunnel: w517 -> [w519 _]
                  frame condition #0 (active) {
                    # "If the module is running standalone, then pop up an error dialog and call the \"Exit\" message."
                    n185 = call <vilib>:"Simple Error Handler.vi"("error in (no error)"=w519) -> ()  [unwired: 4 in, 5 out]
                  }
                  frame condition #1 {
                    # "To prevent the Simple Error Handler VI from being loaded (e.g. when deploying to a Real-Time target), add the Conditional Disable Symbol \"DQMH_Disable_SEH\" to your project and set it to TRUE."
                  }
                }
                n186 = call-poly <vilib>:"Delacor_lib_QMH_Enqueue Message (poly).vi"("Priority Message? (F)"=TRUE, "Message"="Exit", "Message Queue in"=w516) -> ("error out"=w518:errorcluster)  [unwired: 7 in, 1 out]
              }
              frame True {
                # "If the module was launched externally, calling the Error Reported broadcast VI is the only action performed by the \"Error\" message. The module's caller can then process the error appropriately."
              }
            }
            n187 = Merge Errors(w511, w510) -> (w509:errorcluster)
          }
          frame "Write Pump RPM" {
            # "Check auto is not \nrunning"
            # "Checks if the pump is ready"
            # "Writes the pump rpm to the pump drive"
            n188 = local read "EtherCAT System State Out"() -> (w525:map{string, dbl})
            n189 = Look In Map(map=w525, key="Pump Switch on") -> (value=w523:dbl)  [unwired: 1 in, 1 out]
            n190 = call "Check Idle State.vi"() -> ("Idle"=w520:bool)  [unwired: 9 in, 2 out]
            n191 = Not Equal To 0?(x=w523) -> (x != 0?=w521:bool)
            n192 = And(x=w521, y=w520) -> (x .and. y?=w522:bool)
            n193 = case shown="True" w522 {
              frame False {
              }
              frame True {
                # "Sets the rpm"
                # "Enables the pump"
                n194 = call "Write U16.vi"("Variable"="Control Word", "Drive"="Pump", "Data"=u16 15) -> ("error out"=w529:errorcluster)  [unwired: 7 in, 1 out]
                n195 = call "Write Pump RPM.vi"("error in"=w529, "RPM"="Pump Target RPM") -> ()  [unwired: 8 in, 2 out]
              }
            }
          }
          frame "Write Turbine RPM" {
            # "Check auto is not \nrunning"
            # "Checks if the turbine is ready"
            n196 = local read "EtherCAT System State Out"() -> (w537:map{string, dbl})
            n197 = Look In Map(map=w537, key="Turbine Switch on") -> (value=w536:dbl)  [unwired: 1 in, 1 out]
            n198 = call "Check Idle State.vi"() -> ("Idle"=w535:bool)  [unwired: 9 in, 2 out]
            n199 = Not Equal To 0?(x=w536) -> (x != 0?=w534:bool)
            n200 = And(x=w534, y=w535) -> (x .and. y?=w533:bool)
            n201 = case shown="True" w533 {
              frame False {
              }
              frame True {
                # "Sets the turbine rpm"
                # "Enables the turbine"
                n202 = call "Write U16.vi"("Variable"="Control Word", "Drive"="Turbine", "Data"=u16 15) -> ("error out"=w542:errorcluster)  [unwired: 7 in, 1 out]
                n203 = call "Write Turbine RPM.vi"("error in"=w542, "RPM"="Turbine Target RPM") -> ()  [unwired: 8 in, 2 out]
              }
            }
          }
          frame "Write Both RPM" {
            # "Check auto is not \nrunning"
            n204 = local read "EtherCAT System State Out"() -> (w550:map{string, dbl})
            n205 = Look In Map(map=w550, key="Pump Switch on") -> (value=w553:dbl)  [unwired: 1 in, 1 out]
            n206 = Look In Map(map=w550, key="Turbine Switch on") -> (value=w554:dbl)  [unwired: 1 in, 1 out]
            n207 = call "Check Idle State.vi"() -> ("Idle"=w549:bool)  [unwired: 9 in, 2 out]
            n208 = Not Equal To 0?(x=w553) -> (x != 0?=w547:bool)
            n209 = Not Equal To 0?(x=w554) -> (x != 0?=w548:bool)
            n210 = Compound Arithmetic op=AND(w548, w547, w549) -> (w546:bool)
            n211 = case shown="True" w546 {
              frame False {
              }
              frame True {
                # "Sets the turbine rpm"
                # "Enables the turbine"
                # "Sets the turbine rpm"
                # "Enables the turbine"
                n212 = call "Write U16.vi"("wait for reply (T)"=FALSE, "Variable"="Control Word", "Drive"="Turbine", "Data"=u16 15) -> ("error out"=w564:errorcluster)  [unwired: 6 in, 1 out]
                n213 = call "Write U16.vi"("wait for reply (T)"=FALSE, "Variable"="Control Word", "Drive"="Pump", "Data"=u16 15) -> ("error out"=w561:errorcluster)  [unwired: 6 in, 1 out]
                n214 = local read "Pump Target RPM"() -> (w562:i16)
                n215 = local read "Turbine Target RPM"() -> (w563:i16)
                n216 = call "Write Pump RPM.vi"("wait for reply (T)"=FALSE, "error in"=w561, "RPM"=w562) -> ()  [unwired: 7 in, 2 out]
                n217 = call "Write Turbine RPM.vi"("wait for reply (T)"=FALSE, "error in"=w564, "RPM"=w563) -> ()  [unwired: 7 in, 2 out]
              }
            }
          }
          frame "Stop Both Pumps" {
            # "Stops the auto mode sequence"
            # "Disables the Pump"
            # "Disables the turbine"
            n218 = call "Stop Drives.vi"("wait for reply (T)"=FALSE) -> ()  [unwired: 9 in, 2 out]
            n219 = call "Stop Sequence.vi"() -> ()  [unwired: 10 in, 2 out]
          }
          frame "Exit" {
            w588 = 91  # 91: not all Exit messages will have an argument
            w590 = TRUE  # Stop the VI
            # "Release the message queue reference"
            # "#CodeNeeded - Add any required cleanup code here."
            # "Exit - Exit the application."
            n220 = Variant To Data(error in=w598, type=T10 {"Origin"="", "Exit via Stop Module Req?"=FALSE, "Wait for Module to stop?"=FALSE} ("Stop Argument"), Variant=w589) -> (data=w586:T10, error out=w595:errorcluster)
            n221 = call <vilib>:"Clear Errors.vi"("error in (no error)"=w595, "specific error code to clear (0: all)"=w588) -> ("error out"=w597:errorcluster)  [unwired: 4 in, 1 out]
            n222 = control-ref of="This VI"() -> (w585:refnum<vi>)
            n223 = call-dynamic "Delacor_lib_QMH_Release Message Queue.vi"("error in"=w597, "Message Queue"=w592) -> ("error out"=w596:errorcluster)  [unwired: 9 in]
            n224 = call "Handle Exit.vi"("Stop Argument"=w586, "Admin in"=w584, "VI reference"=w585) -> ("error out"=w594:errorcluster)  [unwired: 7 in, 1 out]
            n225 = Merge Errors(w596, w594) -> (w593:errorcluster)
            n226 = call "Error Reported.vi"("Error"=w593) -> ()  [unwired: 10 in, 1 out]
            n227 = local write "error out"(errorcluster {"status"=FALSE, "code"=0, "source"=""} ("error out")) -> ()
            n228 = local write "Pump RPMs"(i64[] []) -> ()
            n229 = local write "Turbine RPMs"(i64[] []) -> ()
            n230 = local write "Duration"(i64[] []) -> ()
            n231 = local write "EtherCAT Connection Status"(FALSE ("EtherCAT Connection Status")) -> ()
            n232 = local write "Current Step"(0 ("Current Step")) -> ()
            n233 = local write "Total Steps"(0 ("Total Steps")) -> ()
            n234 = local write "IOLink Connection Status"(FALSE ("Attempt EtherCAT Connection")) -> ()
            n235 = call "Stop Module.vi"() -> ()  [unwired: 11 in, 1 out]
            n236 = local write "Attempt EtherCAT Connection"(FALSE ("Attempt EtherCAT Connection")) -> ()
            n237 = call "Stop Module.vi"() -> ()  [unwired: 11 in, 1 out]
            n238 = call "Stop Module.vi"() -> ()  [unwired: 11 in, 1 out]
            n239 = local write "System Fault"(FALSE ("System Fault")) -> ()
          }
          frame "Start Logging" {
            n240 = call "Check Idle State.vi"() -> ("Idle"=w602:bool)  [unwired: 9 in, 2 out]
            n241 = case shown="True" w602 {
              tunnel: [_ w604] -> w599
              frame False {
              }
              frame True {
                n242 = call "Create File.vi"("Folder Path"="Folder Path") -> ("error out"=w604:errorcluster)  [unwired: 8 in, 2 out]
              }
            }
            n243 = Merge Errors(w599, w601) -> (w600:errorcluster)
          }
          frame "Stop Logging" {
            n244 = call "Check Idle State.vi"() -> ("Idle"=w606:bool)  [unwired: 9 in, 2 out]
            n245 = case shown="True" w606 {
              frame False {
              }
              frame True {
                n246 = call "Close File.vi"() -> ()  [unwired: 9 in, 3 out]
              }
            }
          }
          frame Default {
            # "'Default' case only runs if there is a message that isn't defined in any of the other cases.  Output a programming error."
            n247 = call "Module Name--constant.vi"() -> ("Module Name"=w613:string)  [unwired: 11 in]
            n248 = Format Into String(format string="The invalid message string \"%s\" was received in the Message Handling Loop for module \"%s\".", w614, w613) -> (resulting string=w609:string)  [unwired: 2 in, 1 out]
            n249 = call <vilib>:"Error Cluster From Error Code.vi"("show call chain? (False)"=TRUE, "error message (\"\")"=w609, "error code (0)"=1) -> ("error out"=w616:errorcluster)  [unwired: 6 in]
            n250 = Merge Errors(w617, w616) -> (w618:errorcluster)
          }
        }
        n251 = call-dynamic "Delacor_lib_QMH_Error Handler - Message Handling Loop.vi"("error in"=w412, "Message Queue in"=w401) -> ("dup error in"=w409:errorcluster)  [unwired: 8 in, 1 out]
      }
      n252 = while {
        tunnel: w41 -> [w270]
        shift-right: [w273] -> w44
        shift-left: w42 -> [w274]
        tunnel: [w275] -> w46
        tunnel: w40 -> [w271]
        stop <- w272 stop-if-true
        # "Event Handling Loop"
        n253 = event "DQMH_EVENT_MAIN" shown="[27] <Auto Modo Broadcast Events.Current RPM Index>: User Event" {
          selector: w274 -> [_ _ _ _ _ _ _ _ w331 _ _ _ _ _ _ _ _ _ _ _ _ _ w377 _ _ w389 _ _ _ _ _ _]
          dyn-events: [_ _ _ _ _ _ _ _ w330 _ _ _ _ _ _ _ _ _ _ _ _ _ w376 _ _ w388 _ _ _ _ _ _] -> w273
          timeout: _ -> [_ _ _ _ _ _ _ _ _ _ _ _ _ _ _ _ _ _ _ _ _ _ _ _ _ _ _ _ _ _ _ _]
          tunnel: [_ _ _ _ _ _ TRUE ("Discard?") _ _ _ _ _ _ _ _ _ _ _ _ _ _ _ _ _ _ _ _ _ _ _ _ _] -> w272
          tunnel: w270 -> [_ w284 _ _ _ _ w308 w315 _ w334 w336 w344 _ w348 w351 w354 w356 w358 w361 w365 _ w371 _ w380 w383 _ w392 _ _ _ _ _]
          tunnel: [w282 w285 _ _ w291 _ w311 w317 w327 w333 _ w343 _ w347 w350 w353 w357 w359 w362 w366 w368 w370 _ w379 w382 _ w391 _ _ _ _ _] -> w276
          tunnel: w271 -> [_ _ _ _ _ _ _ w314 _ _ _ _ _ _ _ _ _ _ _ _ _ _ _ _ _ _ _ _ _ _ _ _]
          event "Simulate EHL Error": Value Change {
            # "#DQMH_HowTo The 'Simulate EHL Error' button  illustrates how the EHL handles errors. This event is instructional in nature and can be removed."
            # "This case simulates an error being generated by the EHL"
            n254 = event-data() -> ()  [unwired: 1 in, 1 out]
            n255 = call "Module Name--constant.vi"() -> ("Module Name"=w279:string)  [unwired: 11 in]
            n256 = Format Into String(format string="Simulated error originating at Event Handling Loop in %s", w279) -> (resulting string=w280:string)  [unwired: 2 in, 1 out]
            n257 = call <vilib>:"Error Cluster From Error Code.vi"("show call chain? (False)"=TRUE, "error message (\"\")"=w280, "error code (0)"=5000) -> ("error out"=w282:errorcluster)  [unwired: 6 in]
          }
          event "Simulate MHL Error": Value Change {
            # "#DQMH_HowTo The 'Simulate MHL Error' button  illustrates how the MHL handles errors. This event is instructional in nature and can be removed."
            # "This case simulates an error being generated by the MHL"
            n258 = event-data() -> ()  [unwired: 1 in, 1 out]
            n259 = call-poly <vilib>:"Delacor_lib_QMH_Enqueue Message (poly).vi"("Message"="Simulate MHL Error", "Message Queue in"=w284) -> ("error out"=w285:errorcluster)  [unwired: 8 in, 1 out]
          }
          event User Event {
            # "Show the panel of this VI, and send a status updated message to let listeners know."
            # "Another Module called the \"Show Panel\" API Method."
            n260 = event-data() -> ()  [unwired: 1 in, 1 out]
            n261 = control-ref of="This VI"() -> (w287:refnum<vi>)
            n262 = call "Open VI Panel.vi"("VI"=w287) -> ()  [unwired: 10 in, 1 out]
            n263 = call "Status Updated.vi"("Status"="Panel shown." ("format string")) -> ()  [unwired: 10 in, 1 out]
          }
          event User Event {
            # "Hide the panel of this VI, and send a status updated message to let listeners know."
            # "Another Module called the \"Hide Panel\" API Method."
            n264 = event-data() -> ()  [unwired: 1 in, 1 out]
            n265 = control-ref of="This VI"() -> (w289:refnum<vi>)
            n266 = call "Hide VI Panel.vi"("VI"=w289) -> ()  [unwired: 10 in, 1 out]
            n267 = call "Status Updated.vi"("Status"="Panel hidden." ("format string")) -> ()  [unwired: 10 in, 1 out]
          }
          event User Event {
            # "Another Module called the \"Get Module Execution Status\" API Method."
            n268 = event-data() -> ()  [unwired: 1 in, 1 out]
            n269 = call "Update Module Execution Status.vi"("Running?"=TRUE) -> ("error out"=w291:errorcluster)  [unwired: 10 in]
          }
          event User Event {
            # "Another Module called the \"Show Diagram\" API Method. This event is used for debugging."
            n270 = event-data() -> ()  [unwired: 1 in, 1 out]
            n271 = disable-structure shown="RUN_TIME_ENGINE==False" {
              frame condition #0 (active) {
                # "functionality not available in exe"
                n272 = invoke class="VI" method="Lock State.Get"() -> (error out=w297:errorcluster, "Get Lock State"=w296:T9, "pwd in cache"=w293:bool)  [unwired: 4 in, 1 out]
                n273 = Equal?(x=T9."Password-protected", y=w296) -> (x = y?=w294:bool)
                n274 = Compound Arithmetic op=AND(w294, invert w293) -> (w292:bool)
                n275 = case shown="False" w292 {
                  tunnel: w297 -> [w300 _]
                  frame False {
                    n276 = property class="VI"(error in=w300, "BDWin.Open"=TRUE ("Block Diagram Window:Open")) -> ()  [unwired: 1 in, 2 out]
                    n277 = call "Status Updated.vi"("Status"="Block Diagram shown." ("format string")) -> ()  [unwired: 10 in, 1 out]
                  }
                  frame True {
                    # "Password-protected VI, and the password is not in the cache. Do not show the diagram."
                  }
                }
              }
              frame condition #1 {
              }
            }
          }
          event User Event {
            # "The Stop Module Event can get fired from the Exit message in the MHL. The queue gets destroyed in that case. If the queue no longer exists, the Enqueue Exit as a priority message will return error 1. It is safe to ignore, because the module is already exiting."
            # "Another Module called the \"Stop Module\" API Method  or the Message Handling Loop below."
            n278 = event-data() -> ("Origin"=w307:string, "Exit via Stop Module Req?"=w303:bool, "Wait for Module to stop?"=w302:bool)  [unwired: 1 in]
            n279 = local write "Status"(w307) -> ()
            n280 = Bundle By Name(cluster=T10 {"Origin"="", "Exit via Stop Module Req?"=FALSE, "Wait for Module to stop?"=FALSE} ("Stop Argument"), "Exit via Stop Module Req?"=w303, "Wait for Module to stop?"=w302) -> (w301:T10)
            n281 = call-poly <vilib>:"Delacor_lib_QMH_Enqueue Message (poly).vi"("Priority Message? (F)"=TRUE, "Message Data"=w301, "Message"="Exit", "Message Queue in"=w308) -> ("error out"=w312:errorcluster)  [unwired: 6 in, 1 out]
            n282 = call <vilib>:"Clear Errors.vi"("error in (no error)"=w312, "specific error code to clear (0: all)"=1) -> ("error out"=w311:errorcluster)  [unwired: 4 in, 1 out]
          }
          event Panel Close? {
            w316 = TRUE  # Discard the event, the MHL is responsible for closing and stopping this VI.
            # "Hide the panel or send the 'Exit' message if the user clicks the 'X' on the module main VI panel."
            n283 = event-data() -> ()  [unwired: 1 in, 1 out]
            n284 = property class="Module Admin"(reference=w314) -> ("Accessors:External Launch"=w313:bool)  [unwired: 1 in, 2 out]
            n285 = case shown="False" w313 {
              tunnel: w315 -> [_ w323]
              tunnel: [_ w324] -> w317
              frame True {
                # "If externally launched, clicking the 'X' hides the panel, but doesn't close it."
                n286 = control-ref of="This VI"() -> (w320:refnum<vi>)
                n287 = call "Hide VI Panel.vi"("VI"=w320) -> ("error out"=w318:errorcluster)  [unwired: 10 in]
                n288 = call "Status Updated.vi"("error in"=w318, "Status"="Panel hidden." ("format string")) -> ()  [unwired: 9 in, 1 out]
              }
              frame False {
                # "If run as a stand-alone VI, clicking the panel 'X' stops the VI."
                n289 = call-poly <vilib>:"Delacor_lib_QMH_Enqueue Message (poly).vi"("Priority Message? (F)"=TRUE, "Message"="Exit", "Message Queue in"=w323) -> ("error out"=w324:errorcluster)  [unwired: 7 in, 1 out]
              }
            }
            n290 = event-data("Discard?"=w316) -> ()  [unwired: 1 in, 1 out]
          }
          event User Event {
            # "This module called the \"Private.Launch Hardware Controller\" private request."
            n291 = event-data() -> ()  [unwired: 1 in, 1 out]
            n292 = call "Start Module.vi"() -> ("error out"=w325:errorcluster, "Wait for Event Sync?"=w328:bool, "Hardware Controller Broadcast Events"=w329:T4)  [unwired: 8 in, 1 out]
            n293 = register-events(reference=w331, error in=w325, w329) -> (reference out=w330:refnum<event-registration>, error out=w326:errorcluster)  [unwired: 3 in]
            n294 = call "Synchronize Module Events.vi"("error in"=w326, "Wait for Event Sync?"=w328) -> ("error out"=w327:errorcluster)  [unwired: 9 in]
          }
          event User Event {
            n295 = event-data() -> ()  [unwired: 1 in, 1 out]
            n296 = call-poly <vilib>:"Delacor_lib_QMH_Enqueue Message (poly).vi"("Message"="Setup Hardware Controller", "Message Queue in"=w334) -> ("error out"=w333:errorcluster)  [unwired: 8 in, 1 out]
          }
          event User Event {
            # "This updates the connection status"
            n297 = event-data() -> ("EtherCAT Connection Status"=w335:bool)  [unwired: 1 in]
            "EtherCAT Connection Status" <- w335
            n298 = case shown="True" w335 {
              tunnel: w336 -> [_ w341]
              tunnel: [errorcluster {"status"=FALSE, "code"=0, "source"=""} ("error out") w340] -> _
              frame False {
              }
              frame True {
                n299 = call-poly <vilib>:"Delacor_lib_QMH_Enqueue Message (poly).vi"("Message"="Get Drive Ready", "Message Queue in"=w341) -> ("error out"=w340:errorcluster)  [unwired: 8 in, 1 out]
                n300 = local write "Attempt EtherCAT Connection"(FALSE ("Attempt EtherCAT Connection")) -> ()
              }
            }
          }
          event "Set Ready": Value Change {
            n301 = event-data() -> ()  [unwired: 1 in, 1 out]
            n302 = call-poly <vilib>:"Delacor_lib_QMH_Enqueue Message (poly).vi"("Message"="Get Drive Ready", "Message Queue in"=w344) -> ("error out"=w343:errorcluster)  [unwired: 8 in, 1 out]
          }
          event User Event {
            n303 = event-data() -> ("Connection State"=→"IOLink Connection Status":bool)  [unwired: 1 in]
          }
          event "Close IOLink Connection": Value Change {
            n304 = event-data() -> ()  [unwired: 1 in, 1 out]
            n305 = call-poly <vilib>:"Delacor_lib_QMH_Enqueue Message (poly).vi"("Message"="Close IOLink Connection", "Message Queue in"=w348) -> ("error out"=w347:errorcluster)  [unwired: 8 in, 1 out]
          }
          event "Load Configuration": Value Change {
            n306 = event-data() -> ()  [unwired: 1 in, 1 out]
            n307 = call-poly <vilib>:"Delacor_lib_QMH_Enqueue Message (poly).vi"("Message"="Load Auto Configuration", "Message Queue in"=w351) -> ("error out"=w350:errorcluster)  [unwired: 8 in, 1 out]
          }
          event "Start EtherCAT Connection": Value Change {
            # "User Operated Start EtherCAT Connection"
            n308 = event-data() -> ()  [unwired: 1 in, 1 out]
            n309 = call-poly <vilib>:"Delacor_lib_QMH_Enqueue Message (poly).vi"("Message"="Start EtherCAT Connection", "Message Queue in"=w354) -> ("error out"=w353:errorcluster)  [unwired: 8 in, 1 out]
          }
          event "Set Pump RPM": Value Change {
            n310 = event-data() -> ()  [unwired: 1 in, 1 out]
            n311 = call-poly <vilib>:"Delacor_lib_QMH_Enqueue Message (poly).vi"("Message"="Write Pump RPM", "Message Queue in"=w356) -> ("error out"=w357:errorcluster)  [unwired: 8 in, 1 out]
          }
          event "Set Turbine RPM": Value Change {
            n312 = event-data() -> ()  [unwired: 1 in, 1 out]
            n313 = call-poly <vilib>:"Delacor_lib_QMH_Enqueue Message (poly).vi"("Message"="Write Turbine RPM", "Message Queue in"=w358) -> ("error out"=w359:errorcluster)  [unwired: 8 in, 1 out]
          }
          event "Set Both RPM": Value Change {
            n314 = event-data() -> ()  [unwired: 1 in, 1 out]
            n315 = call-poly <vilib>:"Delacor_lib_QMH_Enqueue Message (poly).vi"("Message"="Write Both RPM", "Message Queue in"=w361) -> ("error out"=w362:errorcluster)  [unwired: 8 in, 1 out]
          }
          event "Abort": Value Change {
            n316 = event-data() -> ()  [unwired: 1 in, 1 out]
            n317 = call-poly <vilib>:"Delacor_lib_QMH_Enqueue Message (poly).vi"("Message"="Stop Both Pumps", "Message Queue in"=w365) -> ("error out"=w366:errorcluster)  [unwired: 8 in, 1 out]
          }
          event "Close EtherCAT Connection": Value Change {
            # "This closes the EtherCAT Connection"
            n318 = event-data() -> ()  [unwired: 1 in, 1 out]
            n319 = call "Close EtherCAT Connection.vi"("wait for reply (T)"=FALSE) -> ("error out"=w368:errorcluster)  [unwired: 9 in, 1 out]
          }
          event "Start IOLink Connection": Value Change {
            n320 = event-data() -> ()  [unwired: 1 in, 1 out]
            n321 = call-poly <vilib>:"Delacor_lib_QMH_Enqueue Message (poly).vi"("Message"="Start IOLink Connection", "Message Queue in"=w371) -> ("error out"=w370:errorcluster)  [unwired: 8 in, 1 out]
          }
          event User Event {
            # "This module called the \"Private.Start Logger Module\" private request."
            n322 = event-data() -> ()  [unwired: 1 in, 1 out]
            n323 = call "Start Module.vi"() -> ("error out"=w373:errorcluster, "Wait for Event Sync?"=w374:bool, "Logger Broadcast Events"=w375:T2)  [unwired: 8 in, 1 out]
            n324 = register-events(reference=w377, error in=w373, w375) -> (reference out=w376:refnum<event-registration>, error out=w372:errorcluster)  [unwired: 3 in]
            n325 = call "Synchronize Module Events.vi"("error in"=w372, "Wait for Event Sync?"=w374) -> ()  [unwired: 9 in, 1 out]
          }
          event "Start Logging": Value Change {
            n326 = event-data() -> ()  [unwired: 1 in, 6 out]
            n327 = call-poly <vilib>:"Delacor_lib_QMH_Enqueue Message (poly).vi"("Message"="Start Logging", "Message Queue in"=w380) -> ("error out"=w379:errorcluster)  [unwired: 8 in, 1 out]
          }
          event "Stop Logging": Value Change {
            n328 = event-data() -> ()  [unwired: 1 in, 6 out]
            n329 = call-poly <vilib>:"Delacor_lib_QMH_Enqueue Message (poly).vi"("Message"="Stop Logging", "Message Queue in"=w383) -> ("error out"=w382:errorcluster)  [unwired: 8 in, 1 out]
          }
          event User Event {
            # "This module called the \"Private.Start Auto Mode Module\" private request."
            n330 = event-data() -> ()  [unwired: 1 in, 1 out]
            n331 = call "Start Module.vi"() -> ("error out"=w385:errorcluster, "Wait for Event Sync?"=w386:bool, "Auto Modo Broadcast Events"=w387:T3)  [unwired: 8 in, 1 out]
            n332 = register-events(reference=w389, error in=w385, w387) -> (reference out=w388:refnum<event-registration>, error out=w384:errorcluster)  [unwired: 3 in]
            n333 = call "Synchronize Module Events.vi"("error in"=w384, "Wait for Event Sync?"=w386) -> ()  [unwired: 9 in, 1 out]
          }
          event "Start Sequence": Value Change {
            n334 = event-data() -> ()  [unwired: 1 in, 6 out]
            n335 = call-poly <vilib>:"Delacor_lib_QMH_Enqueue Message (poly).vi"("Message"="Start Auto Mode Sequence", "Message Queue in"=w392) -> ("error out"=w391:errorcluster)  [unwired: 8 in, 1 out]
          }
          event User Event {
            n336 = event-data() -> ("Current Index"=w396:i32)  [unwired: 1 in, 4 out]
            n337 = Increment(x=w396) -> (x+1=→"Current Step" →"Steps Slide":i32)
            n338 = local read "Pump RPMs"() -> (w395:i64[])
            n339 = Array Size(array=w395) -> (size(s)=w393:i32)
            "Total Steps" <- w393
            n340 = property on="Steps Slide" class="Slide (strict)"("Scale.Maximum"=w393) -> ()  [unwired: 2 in, 2 out]
          }
          event User Event {
            n341 = event-data() -> ("Logging"=→"Logging":bool)  [unwired: 1 in, 4 out]
          }
          event User Event {
            n342 = event-data() -> ("Auto Mode?"=→"Auto Mode Status":bool)  [unwired: 1 in, 4 out]
          }
          event User Event {
            n343 = event-data() -> ("System Fault"=→"System Fault":bool)  [unwired: 1 in, 4 out]
          }
          event "Clear Fault": Value Change {
            n344 = event-data() -> ()  [unwired: 1 in, 6 out]
            n345 = local write "error out"(errorcluster {"status"=FALSE, "code"=0, "source"=""} ("error out")) -> ()
            n346 = call "Clear System Fault.vi"() -> ()  [unwired: 10 in, 2 out]
          }
        }
        n347 = call-dynamic "Delacor_lib_QMH_Error Handler - Event Handling Loop.vi"("error in"=w276, "Message Queue in"=w270) -> ("dup error in"=w275:errorcluster)  [unwired: 8 in, 1 out]
      }
      n348 = Unregister For Events(event registration refnum=w29) -> ()  [unwired: 1 in, 1 out]
      n349 = Unregister For Events(event registration refnum=w24) -> ()  [unwired: 1 in, 1 out]
      n350 = Unregister For Events(event registration refnum=w34) -> ()  [unwired: 1 in, 1 out]
      n351 = Unregister For Events(event registration refnum=w38) -> ()  [unwired: 1 in, 1 out]
    }
    frame Error {
      # "Synchronize Caller Events.vi will inform Start Module.vi that the module has launched and will let the code calling Start Module.vi register for broadcasts and would permit the caller receive the broadcast that an error occurred at launch time."
      n352 = call-dynamic "Delacor_lib_QMH_Release Message Queue.vi"("error in"=w626, "Message Queue"=w619) -> ("error out"=w625:errorcluster)  [unwired: 9 in]
      n353 = call "Synchronize Caller Events.vi"("Singleton Module Admin in"=w620) -> ("error out"=w627:errorcluster)  [unwired: 9 in, 1 out]
      n354 = call "Module Name--constant.vi"() -> ("Module Name"=w623:string)  [unwired: 11 in]
      n355 = Format Into String(format string="An error occurred during initialization. %s is no longer running.", w623) -> (resulting string=w621:string)  [unwired: 2 in, 1 out]
      n356 = Merge Errors(w625, w627) -> (w628:errorcluster)
      n357 = call "Error Reported.vi"("Additional Information"=w621, "Error"=w628) -> ()  [unwired: 9 in, 1 out]
    }
  }
  n358 = Merge Errors(w17, w20) -> (w16:errorcluster)
  n359 = call "Close Module.vi"("error in"=w16, "Module Admin in"=w12) -> ("error out"=w18:errorcluster, "External Launch"=w6:bool, "Module Admin out"=w7:refnum<class "Delacor_lib_QMH_Module Admin.lvclass">)  [unwired: 7 in]
  n360 = Unregister For Events(event registration refnum=w11, error in=w18) -> (error out=w4:errorcluster)
  "error out" <- w4
  n361 = case "External Launch?" shown="True" w6 {
    tunnel: w4 -> [_ w629]
    frame False {
    }
    frame True {
      n362 = case shown="No Error" w629 {
        frame No Error {
          n363 = invoke class="VI" method="FP.Close"() -> ()  [unwired: 3 in, 3 out]
        }
        frame Error {
          n364 = invoke class="VI" method="FP.Open"("Activate"=TRUE ("Activate?")) -> ()  [unwired: 4 in, 5 out]
        }
      }
    }
  }
  n365 = local write "Module Admin"(w7) -> ()
